vi "datataker.vi"() -> ()   [LabVIEW 2012]
doc: "This example demonstrates how to acquire a single buffer of voltage measurements using a DAQmx device.\n\nFor instructions on how to connect your signals to the DAQ device, refer to your device documentation."
uses:
  <vilib>/userdefined/High Color/nirio_resource_hc.ctl
  <vilib>/Utility/error.llb/DialogType.ctl
  <vilib>/addons/h5labview2/file/H5Fmode.ctl
  <vilib>/DAQmx/read.llb/DAQmx Read (Analog 2D DBL NChan NSamp).vi
  <vilib>/addons/h5labview2/base/lib_path.vi
  <vilib>/DAQmx/read.llb/DAQmx Read (Analog 1D Wfm NChan NSamp).vi
  <vilib>/FPGAPlugInAG/PCIe-7841R/niLvFpga_Open_PCIe-7841R.vi
  <vilib>/DAQmx/create/channels.llb/DAQmx Create Channel (AI-Voltage-Basic).vi
  <vilib>/DAQmx/configure/timing.llb/DAQmx Timing (Sample Clock).vi
  <vilib>/DAQmx/configure/task.llb/DAQmx Configure Logging (TDMS).vi
  <vilib>/DAQmx/configure/trigger.llb/DAQmx Start Trigger (Digital Edge).vi
  <vilib>/DAQmx/configure/trigger.llb/DAQmx Start Trigger (Analog Edge).vi
  <vilib>/DAQmx/configure/trigger.llb/DAQmx Reference Trigger (Digital Edge).vi
  <vilib>/DAQmx/configure/trigger.llb/DAQmx Reference Trigger (Analog Edge).vi
  <vilib>/Utility/error.llb/Error Cluster From Error Code.vi
  <vilib>/rvi/errors/niLvFpgaAdjustHostInterfaceError.vi
  <vilib>/DAQmx/miscellaneous.llb/DAQmx Fill In Error Info.vi
  <vilib>/addons/h5labview2/base/H5Equery.vi
  vis/Multiple Waveforms.vi
  <vilib>/Waveform/WDTFileIO.llb/Export Waveforms To Spreadsheet File (1D).vi
  <vilib>/rvi/interface/nirviOpenFPGA/nirviOpenFPGA.xnode
  vis/FPGA Bitfiles/MultiChannelFeed_FPGATarget2_feedbackcooling(_T5hmXv3JUos.lvbitx
  <vilib>/rvi/interface/nirviReadWriteControl/nirviReadWriteControl.xnode
  <vilib>/addons/h5labview2/dataset/H5Dwrite.llb/H5Dwrite.xnode
  <vilib>/addons/h5labview2/attrib/H5Awrite.llb/H5Awrite.xnode
  <resource>/objmgr/daqmx.rc
  <vilib>/addons/h5labview2/file/H5F.lvlib
  <vilib>/addons/h5labview2/group/H5G.lvlib
  NiFpgaLv.dll
panel:
  in  "File base name":string="charge"
  in  "Delay time between files(s)":dbl caption="Delay Time (s)"
  in  "Num files":i32
  out "Array":dbl[](array[numeric])=[21.8, 23.5]
  in  "VISA Refnum in":refnum<visa-resource-name>="GPIB0::19::INSTR"
  in  "RIO Device":T1="RIO0::INSTR"
  in  "File type":string="Binary"
  in  "Directory path":path=path "D:/Data/20140529/Bead1/1e-2mbar_axcool_41Hzx.h5"
  in  "Trigger Type":T2(tab)
  in  "Edge":i32(ring)=10280 items=["Rising"=10280, "Falling"=10171]
  in  "Digital Trigger Source":tag
  in  "Level (V)":dbl format="%0.2f"
  in  "Hysteresis (V)":dbl
  in  "Slope":i32(ring)=10280 items=["Rising"=10280, "Falling"=10171]
  in  "Analog Trigger Source":string="APFI0"
  in  "Digital Ref Trigger Source":tag
  in  "Edge":i32(ring)=10280 items=["Rising"=10280, "Falling"=10171]
  in  "Pre-Trigger Samples":u32
  in  "Analog Ref Trigger Source":string="APFI0"
  in  "Slope":i32(ring)=10280 items=["Rising"=10280, "Falling"=10171]
  in  "Level (V)":dbl format="%0.2f"
  in  "Pre-Trigger Samples":u32
  out "Waveform Graph":dbl[][](graph)
  in  "TDMS File Path":path
  in  "Number of Samples":i32=150000
  in  "Sample Rate":dbl=15000.0
  in  "Sample Clock Source":tag="OnboardClock"
  in  "Terminal Configuration":i32(ring)=-1 items=["default"=-1, "RSE"=10083, "NRSE"=10078, "Differential"=10106, "Pseudodifferential"=12529]
  in  "Max Voltage":dbl=5.0
  in  "Physical Channel":tag="Dev1/ai0:3"
  out "Actual Sample Rate":dbl=15003.750937734434 format="%0.2f"
  in  "Logging Mode":i32(ring)=10231 items=["Off"=10231, "Log and Read"=15842]
  # "Channel Settings"
  # "Acquired Data"
  # "Timing Settings"
  # "Trigger Settings"
  # "Logging Settings"
  # "To configure and use a start trigger you must have the necessary tab selected above.  Not all hardware supports triggering--refer to your device documentation for more info."
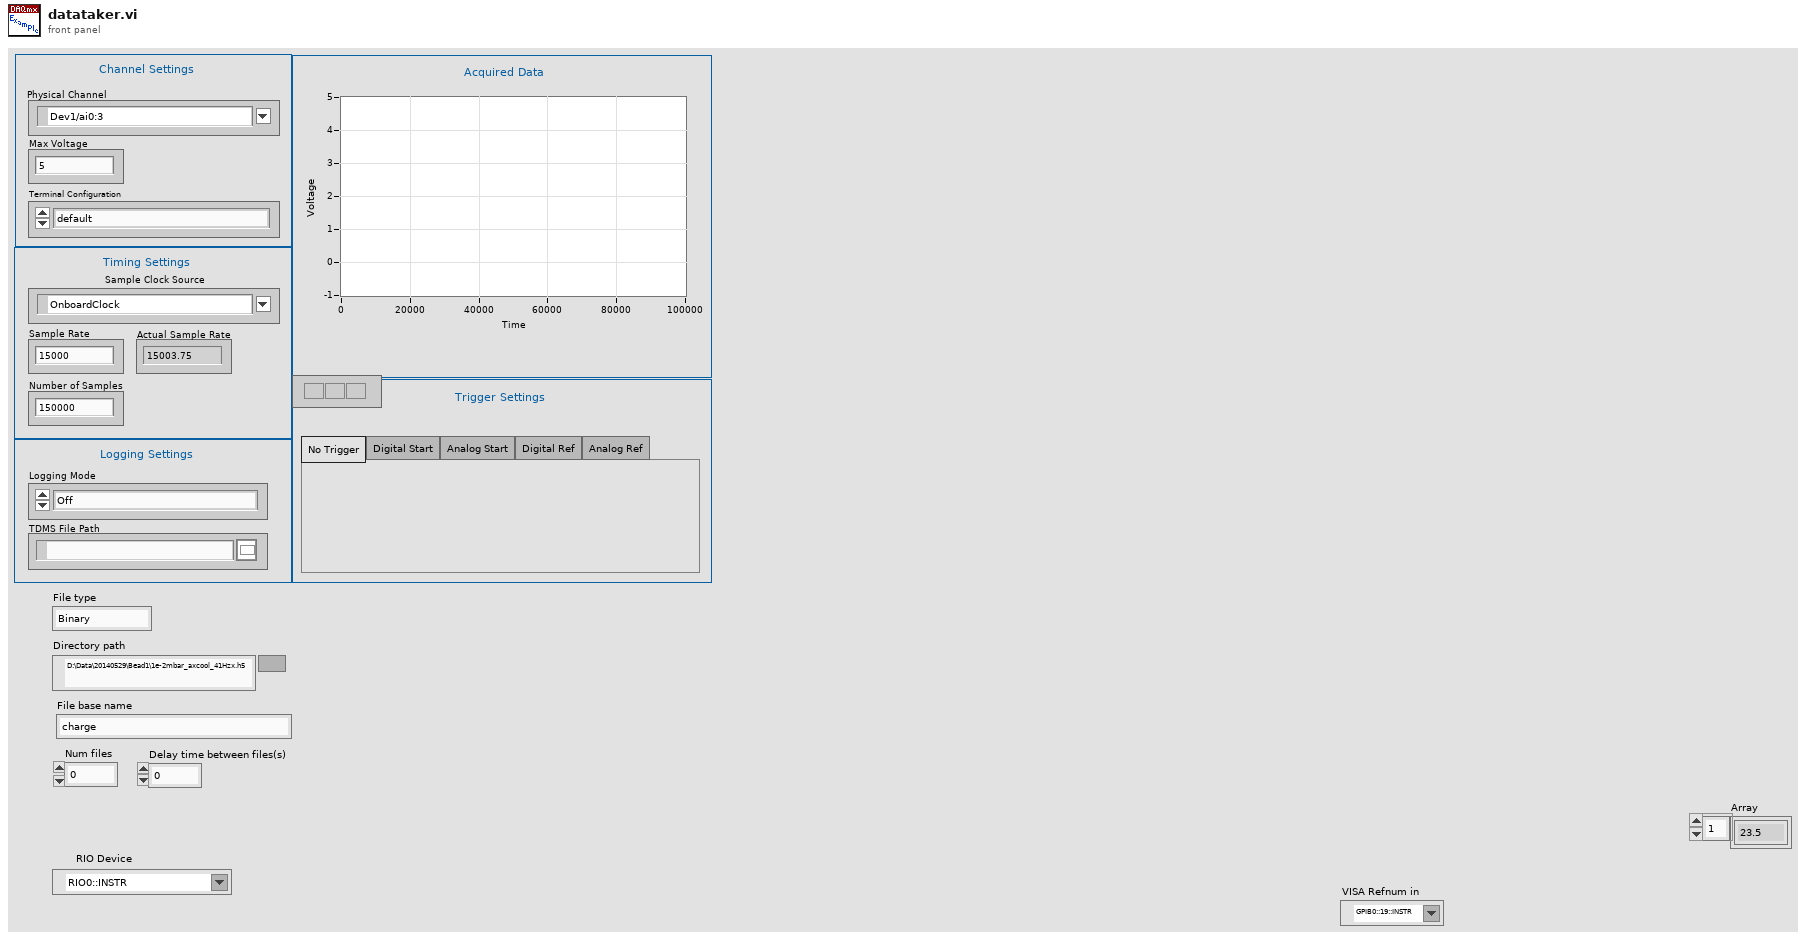
[diagram p1: front panel]
types:
  T1 = typedef "nirio_resource_hc.ctl" = tag
  T2 = enum32{"No Trigger", "Digital Start", "Analog Start", "Digital Ref", "Analog Ref"}
  T3 = typedef "H5F.lvlib/H5Fmode.ctl" = enum16{"read-only", "read-write", "overwrite", "create new", "open or create"}
  T4 = typedef "DialogType.ctl" = u16
  T5 = typedef "hid_t.ctl" = i32
  T6 = cluster{"pg 0":fxp<+/-,32,16>, "dg 0":fxp<+/-,32,16>, "pg 1":fxp<+/-,32,16>, "dg 1":fxp<+/-,32,16>, "pg 2":fxp<+/-,32,16>, "dg 2":fxp<+/-,32,16>, "Dc offset 0":fxp<+/-,32,16>, "Dc offset 1":fxp<+/-,32,16>, "Dc offset 2":fxp<+/-,32,16>}
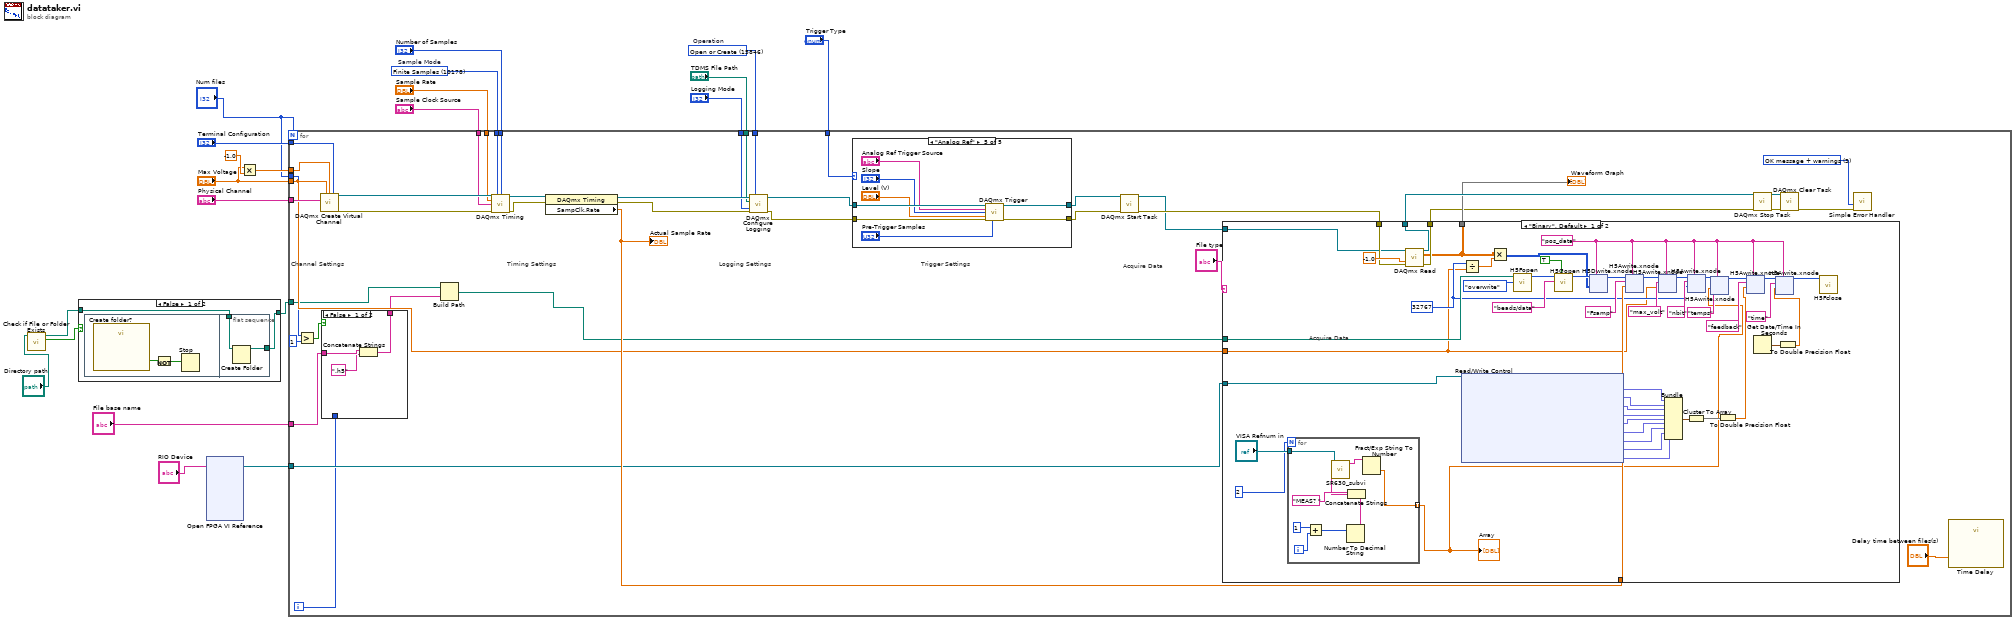
[diagram p0: block diagram]
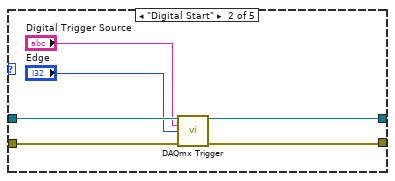
[diagram p4: hidden frame]
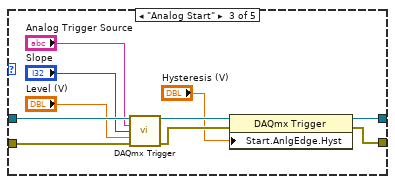
[diagram p5: hidden frame]
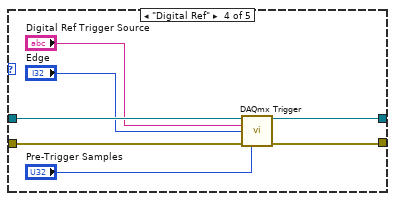
[diagram p6: hidden frame]
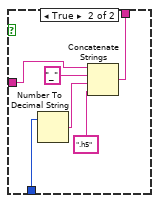
[diagram p7: hidden frame]
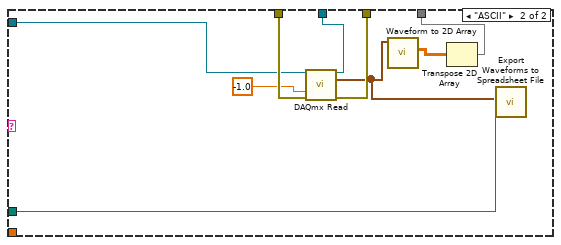
[diagram p8: hidden frame]
diagram:
  w20 = 15846 items=["Open"=10437, "Open or Create"=15846, "Create or Replace"=15847, "Create"=15848]  # Operation
  w21 = 10178 items=["Finite Samples"=10178, "Continuous Samples"=10123, "Hardware Timed Single Point"=12522]  # Sample Mode
  n1 = call <vilib>:"Check if File or Folder Exists.vi"("path"="Directory path") -> ("file or folder exists?"=w6:bool, "dup path"=w5:path)  [unwired: 8 in, 1 out]
  n2 = case shown="False" w6 {
    tunnel: w5 -> [w23 w28]
    tunnel: [w22 w28] -> w4
    frame False {
      n3 = flat-sequence {
        tunnel: w23 -> [w27]
        tunnel: [w26] -> w22
        frame #0 {
          n4 = call "Create folder?"() -> ("OK"=w25:bool)  [unwired: 18 in, 1 out]
          n5 = Not(x=w25) -> (.not. x?=w24:bool)
          n6 = Stop(stop? (T)=w24) -> ()
        }
        frame #1 {
          n7 = Create Folder(path (use dialog)=w27) -> (created path=w26:path)  [unwired: 2 in, 2 out]
        }
      }
    }
    frame True {
    }
  }
  n8 = xnode "Open FPGA VI Reference"("resource name"="RIO Device") -> ("FPGA VI Reference Out"=w8:refnum<k20>)  [unwired: 1 in, 1 out]
  n9 = Multiply(x="Max Voltage", y=-1.0) -> (x*y=w11:dbl)
  n10 = for {
    N: "Num files" -> [_]
    tunnel: w21 -> [w69]
    tunnel: w20 -> [w64]
    tunnel: "Logging Mode" -> [w62]
    tunnel: "Physical Channel" -> [w61]
    tunnel: "Terminal Configuration" -> [w60]
    tunnel: "Sample Clock Source" -> [w59]
    tunnel: "Sample Rate" -> [w58]
    tunnel: "TDMS File Path" -> [w57]
    tunnel: "Number of Samples" -> [w56]
    tunnel: w11 -> [w45]
    tunnel: "Max Voltage" -> [w44]
    tunnel: w8 -> [w43]
    tunnel: w4 -> [w41]
    tunnel: "Num files" -> [w40]
    tunnel: "File base name" -> [w36]
    tunnel: "Trigger Type" -> [w29]
    i -> [w35]
    w53 = T4 3 items=["no dialog", "OK message", "continue or stop message", "OK message + warnings", "continue/stop + warnings"] ("type of dialog (OK msg:1)")
    # "Acquire Data"
    # "Acquire Data"
    # "Trigger Settings"
    # "Timing Settings"
    # "Channel Settings"
    # "Logging Settings"
    n11 = Greater?(x=w40, y=1) -> (0:w38:bool)
    n12 = call-poly <vilib>:"DAQmx Create Virtual Channel.vi"("maximum value"=w44, "minimum value"=w45, "input terminal configuration"=w60, "physical channels"=w61) -> ("task out"=w67:refnum<k21>, "error out"=w68:errorcluster)  [unwired: 10 in]
    n13 = case shown="False" w38 {
      tunnel: w36 -> [w107 w113]
      tunnel: w35 -> [_ w110]
      tunnel: [w105 w108] -> w34
      frame False {
        n14 = Concatenate Strings(w107, ".h5" ("string")) -> (w105:string)
      }
      frame True {
        n15 = Number To Decimal String(number=w110) -> (decimal integer string=w111:string)  [unwired: 1 in]
        n16 = Concatenate Strings(w113, "_" ("string"), w111, ".h5" ("string")) -> (w108:string)
      }
    }
    n17 = Build Path(base path=w41, name or relative path=w34) -> (appended path=w37:path)
    n18 = call-poly <vilib>:"DAQmx Timing.vi"("task/channels in"=w67, "sample mode"=w69, "samples per channel"=w56, "rate"=w58, "source"=w59, "error in"=w68) -> ("task out"=w71:refnum<k21>, "error out"=w70:errorcluster)  [unwired: 8 in]
    n19 = property class="DAQmx Timing"(reference=w71, error in=w70) -> (reference out=w66:refnum<k21>, error out=w65:errorcluster, "SampClk.Rate"=w51:dbl)
    "Actual Sample Rate" <- w51
    n20 = call-poly <vilib>:"DAQmx Configure Logging.vi"("task/channels in"=w66, "operation"=w64, "file path"=w57, "logging mode"=w62, "error in"=w65) -> ("task out"=w33:refnum<k21>, "error out"=w32:errorcluster)  [unwired: 9 in]
    n21 = case shown="\"Analog Ref\"" w29 {
      tunnel: w33 -> [w73 w79 w89 w96 w104]
      tunnel: w32 -> [w72 w78 w88 w95 w103]
      tunnel: [w73 w77 w86 w94 w98] -> w30
      tunnel: [w72 w76 w85 w93 w99] -> w31
      frame "No Trigger", Default {
      }
      frame "Digital Start" {
        n22 = call-poly <vilib>:"DAQmx Trigger.vi"("task/channels in"=w79, "source"="Digital Trigger Source", "edge"="Edge", "error in"=w78) -> ("task out"=w77:refnum<k21>, "error out"=w76:errorcluster)  [unwired: 10 in]
      }
      frame "Analog Start" {
        n23 = call-poly <vilib>:"DAQmx Trigger.vi"("task/channels in"=w89, "source"="Analog Trigger Source", "slope"="Slope", "level"="Level (V)", "error in"=w88) -> ("task out"=w84:refnum<k21>, "error out"=w83:errorcluster)  [unwired: 9 in]
        n24 = property class="DAQmx Trigger"(reference=w84, error in=w83, "Start.AnlgEdge.Hyst"="Hysteresis (V)") -> (reference out=w86:refnum<k21>, error out=w85:errorcluster)
      }
      frame "Digital Ref" {
        n25 = call-poly <vilib>:"DAQmx Trigger.vi"("task/channels in"=w96, "source"="Digital Ref Trigger Source", "edge"="Edge", "error in"=w95, "pretrigger samples per channel"="Pre-Trigger Samples") -> ("task out"=w94:refnum<k21>, "error out"=w93:errorcluster)  [unwired: 9 in]
      }
      frame "Analog Ref" {
        n26 = call-poly <vilib>:"DAQmx Trigger.vi"("task/channels in"=w104, "source"="Analog Ref Trigger Source", "slope"="Slope", "level"="Level (V)", "error in"=w103, "pretrigger samples per channel"="Pre-Trigger Samples") -> ("task out"=w98:refnum<k21>, "error out"=w99:errorcluster)  [unwired: 8 in]
      }
    }
    n27 = call <vilib>:"DAQmx Start Task.vi"("task/channels in"=w30, "error in"=w31) -> ("task out"=w49:refnum<k21>, "error out"=w50:errorcluster)  [unwired: 12 in]
    n28 = case shown="\"Binary\", Default" "File type" {
      tunnel: w37 -> [w162 w306]
      tunnel: w51 -> [w154 _]
      tunnel: w50 -> [w152 w305]
      tunnel: w49 -> [w149 w304]
      tunnel: [w150 w302] -> w48
      tunnel: [w144 w298] -> w47
      tunnel: [w151 w301] -> w46
      tunnel: w44 -> [w141 _]
      tunnel: w43 -> [w117 _]
      frame "Binary", Default {
        w142 = i16 32767 ("y")
        w122 = "pos_data" ("dataset name")
        n29 = for {
          N: 2 ("dimension size") -> [_]
          tunnel: "VISA Refnum in" -> [w171]
          tunnel: [w169] -> w118 mode=indexing
          i -> [w168]
          n30 = Add(x=1, y=w168) -> (x+y=w166:i32)
          n31 = Number To Decimal String(number=w166) -> (decimal integer string=w165:string)  [unwired: 1 in]
          n32 = Concatenate Strings("MEAS? " ("Write Buffer"), w165) -> (w163:string)
          n33 = call "SR630_subvi.vi"("Write Buffer"=w163, "VISA Refnum in"=w171) -> ("read buffer"=w170:string)  [unwired: 9 in]
          n34 = Fract/Exp String To Number(string=w170) -> (number=w169:dbl)  [unwired: 3 in, 1 out]
        }
        "Array" <- w118
        n35 = call-poly <vilib>:"DAQmx Read.vi"("task/channels in"=w149, "timeout"=-1.0, "error in"=w152) -> ("task out"=w150:refnum<k21>, "data"=w144:dbl[][], "error out"=w151:errorcluster)  [unwired: 10 in]
        n36 = xnode "Read/Write Control"("FPGA VI Reference In"=w117) -> ("pg 0"=w134:fxp<+/-,32,16>, "dg 0"=w133:fxp<+/-,32,16>, "pg 1"=w132:fxp<+/-,32,16>, "dg 1"=w131:fxp<+/-,32,16>, "pg 2"=w130:fxp<+/-,32,16>, "dg 2"=w129:fxp<+/-,32,16>, "Dc offset 0"=w128:fxp<+/-,32,16>, "Dc offset 1"=w127:fxp<+/-,32,16>, "Dc offset 2"=w126:fxp<+/-,32,16>)  [unwired: 1 in, 2 out]
        n37 = Divide(x=w142, y=w141) -> (x/y=w143:dbl)
        n38 = Multiply(x=w144, y=w143) -> (x*y=w140:i16[][])
        n39 = call <vilib>:"H5Fopen.vi"("mode (read-only)"=H5Fmode."overwrite", "path"=w162) -> ("ref out"=w158:T5)  [unwired: 2 in, 1 out]
        n40 = call <vilib>:"H5Gopen.vi"("create? (F)"=TRUE, "name"="beads/data", "ref in"=w158) -> ("group out"=w157:T5)  [unwired: 4 in, 1 out]
        n41 = xnode "H5Dwrite.xnode"("dataset name"=w122, "data"=w140, "ref in"=w157) -> ("ref out"=w156:i32)  [unwired: 4 in, 2 out]
        n42 = xnode "H5Awrite.xnode"("object name"=w122, "data"=w154, "attrib name"="Fsamp", "ref in"=w156) -> ("ref out"=w148:i32)  [unwired: 3 in, 2 out]
        n43 = xnode "H5Awrite.xnode"("object name"=w122, "data"=w141, "attrib name"="max_volt", "ref in"=w148) -> ("ref out"=w146:i32)  [unwired: 3 in, 2 out]
        n44 = Bundle("pg 0"=w134, "dg 0"=w133, "pg 1"=w132, "dg 1"=w131, "pg 2"=w130, "dg 2"=w129, "Dc offset 0"=w128, "Dc offset 1"=w127, "Dc offset 2"=w126) -> (w135:T6)  [unwired: 1 in]
        n45 = xnode "H5Awrite.xnode"("object name"=w122, "data"=w142, "attrib name"="nbit", "ref in"=w146) -> ("ref out"=w138:i32)  [unwired: 3 in, 2 out]
        n46 = Cluster To Array(cluster=w135) -> (array=w125:fxp<+/-,32,16>[])
        n47 = xnode "H5Awrite.xnode"("object name"=w122, "data"=w118, "attrib name"="temps", "ref in"=w138) -> ("ref out"=w137:i32)  [unwired: 3 in, 2 out]
        n48 = To Double Precision Float(number=w125) -> (double precision float=w124:dbl[])
        n49 = xnode "H5Awrite.xnode"("object name"=w122, "data"=w124, "attrib name"="feedback", "ref in"=w137) -> ("ref out"=w121:i32)  [unwired: 3 in, 2 out]
        n50 = Get Date/Time In Seconds() -> (seconds since 1Jan1904=w116:timestamp)
        n51 = To Double Precision Float(number=w116) -> (double precision float=w115:dbl)
        n52 = xnode "H5Awrite.xnode"("object name"=w122, "data"=w115, "attrib name"="time", "ref in"=w121) -> ("ref out"=w114:i32)  [unwired: 3 in, 2 out]
        n53 = call <vilib>:"H5Fclose.vi"("ref"=w114) -> ()  [unwired: 4 in, 1 out]
      }
      frame "ASCII" {
        n54 = call-poly <vilib>:"DAQmx Read.vi"("task/channels in"=w304, "timeout"=-1.0, "error in"=w305) -> ("task out"=w302:refnum<k21>, "data"=w300:waveform(dbl)[], "error out"=w301:errorcluster)  [unwired: 10 in]
        n55 = call-poly "Waveform to 2D Array.vi"("Multiple Waveforms"=w300) -> ("2D Array"=w299:dbl[][])  [unwired: 9 in, 1 out]
        n56 = Transpose 2D Array(2D array=w299) -> (transposed array=w298:dbl[][])
        n57 = call-poly <vilib>:"Export Waveforms to Spreadsheet File.vi"("waveforms"=w300, "file path (dialog if empty)"=w306) -> ()  [unwired: 8 in, 2 out]
      }
    }
    "Waveform Graph" <- w47
    n58 = call <vilib>:"DAQmx Stop Task.vi"("task/channels in"=w48, "error in"=w46) -> ("task out"=w55:refnum<k21>, "error out"=w54:errorcluster)  [unwired: 12 in]
    n59 = call <vilib>:"DAQmx Clear Task.vi"("task in"=w55, "error in"=w54) -> ("error out"=w63:errorcluster)  [unwired: 13 in]
    n60 = call <vilib>:"Simple Error Handler.vi"("type of dialog (OK msg:1)"=w53, "error in (no error)"=w63) -> ()  [unwired: 3 in, 5 out]
    n61 = call "Time Delay"("Delay Time (s)"="Delay time between files(s)") -> ()  [unwired: 10 in, 1 out]
  }
